vi "Kxx_Kxy_calc.vi"(5 "Sample_w":dbl, 6 "HTR Power":dbl, 7 "Sample_t":dbl, 8 "dTxy":dbl, 9 "dTxx":dbl, 10 "Sample_Lxx":dbl, 11 "Sample_Lxy":dbl) -> (2 "Kxx":dbl, 3 "Kxy":dbl)   [LabVIEW 2023]
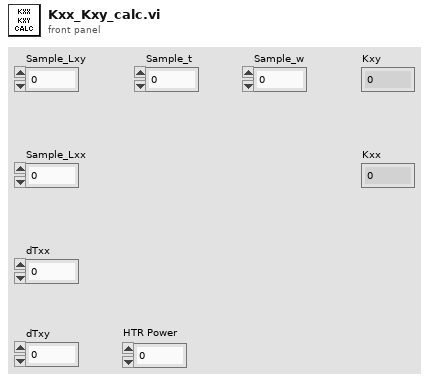
[diagram p1: front panel]
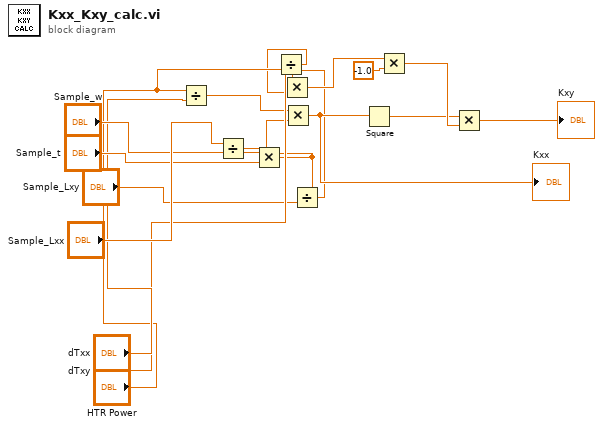
[diagram p0: block diagram]
diagram:
  n1 = Divide(x="HTR Power", y="dTxx") -> (x/y=w2:dbl)
  n2 = Multiply(x="Sample_w", y="Sample_t") -> (x*y=w3:dbl)
  n3 = Divide(x="Sample_Lxx", y=w3) -> (x/y=w1:dbl)
  n4 = Divide(x="dTxy", y="HTR Power") -> (x/y=w6:dbl)
  n5 = Multiply(x=w2, y=w1) -> (x*y=w9:dbl)
  "Kxx" <- w9
  n6 = Divide(x=w3, y="Sample_Lxy") -> (x/y=w5:dbl)
  n7 = Multiply(x=w5, y=w6) -> (x*y=w7:dbl)
  n8 = Square(x=w9) -> (x^2=w8:dbl)
  n9 = Multiply(x=w7, y=-1.0) -> (x*y=w10:dbl)
  n10 = Multiply(x=w8, y=w10) -> (x*y=→"Kxy":dbl)
